vi "markReadOnly.vi"(8 "error in (no error)":errorcluster, 11 "Context in":T1) -> (0 "error out":errorcluster, 3 "Context out":T1)   [LabVIEW 2022 SP3, in "Property Editor.lvlib"]
uses:
  Property Editor.lvlib
  Public/Classes/IComponent/IComponent.lvclass
  TypeDef/DisplayType.ctl
  TypeDef/Context.ctl
  Public/Classes/IProperty/IProperty.lvclass
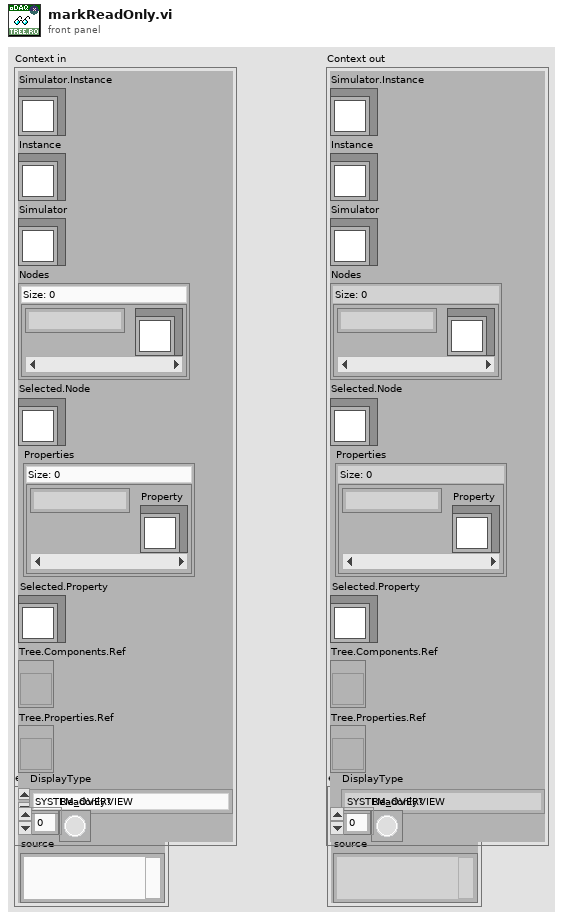
[diagram p1: front panel]
types:
  T1 = typedef "Property Editor.lvlib/Context.ctl" = cluster{"Simulator.Instance":refnum<class "IComponent.lvclass">, "Instance":refnum<class "IComponent.lvclass">, "Simulator":refnum<class "IComponent.lvclass">, "Nodes":map{string, refnum<class "IComponent.lvclass">}, "Selected.Node":refnum<class "IComponent.lvclass">, "Properties":map{string, refnum<class "IProperty.lvclass">}, "Selected.Property":refnum<class "IProperty.lvclass">, "Tree.Components.Ref":refnum<vi>, "Tree.Properties.Ref":refnum<vi>, "DisplayType":T2, "Readonly?":bool[]}
  T2 = typedef "Property Editor.lvlib/DisplayType.ctl" = enum16{"SYSTEM_OVERVIEW", "SIGNALS", "CHANNELS", "FUNCTION_BLOCKS", "TOPOLOGY", "TOPOLOGY_CUSTOM_COMPONENTS", "UNSPECIFIED"}
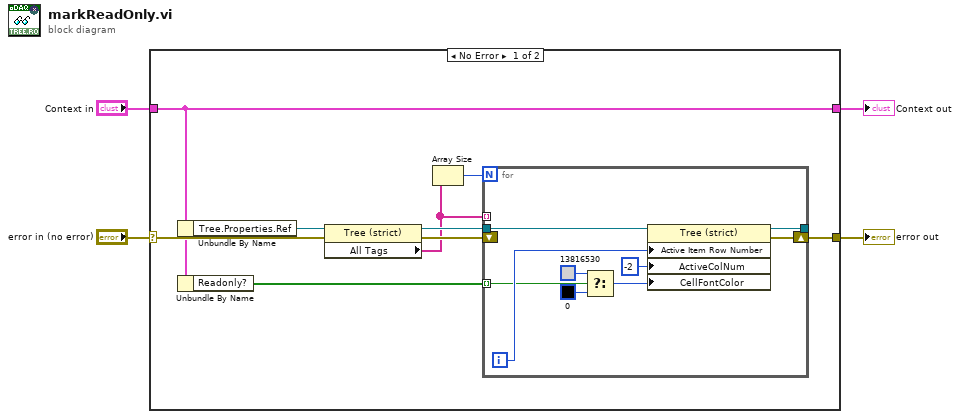
[diagram p0: block diagram]
diagram:
  n1 = case shown="No Error" "error in (no error)" {
    selector: "error in (no error)" -> [w8 w24]
    tunnel: [w13 w24] -> w4
    tunnel: "Context in" -> [w5 w23]
    tunnel: [w5 w23] -> w1
    frame No Error {
      n2 = Unbundle By Name(w5) -> ("Tree.Properties.Ref"=w7:refnum<vi>)
      n3 = Unbundle By Name(w5) -> ("Readonly?"=w6:bool[])
      n4 = property class="Tree (strict)"(reference=w7, error in=w8) -> (reference out=w11:refnum<vi>, error out=w12:errorcluster, "All Tags"=w10:string[])
      n5 = Array Size(array=w10) -> (size(s)=w9:i32)
      n6 = for {
        N: w9 -> [_]
        tunnel: w11 -> [w21]
        tunnel: w10 -> [_] mode=indexing
        tunnel: [w16] -> _
        shift-right: [w15] -> w13
        shift-left: w12 -> [_]
        tunnel: w6 -> [w14] mode=indexing
        i -> [w20]
        n7 = Select(t=u32 13816530 ("Active Cell:Cell Font:Color"), s=w14, f=u32 0 ("Active Cell:Cell Font:Color")) -> (s? t:f=w17:u32)
        n8 = property class="Tree (strict)"(reference=w21, "Active Item Row Number"=w20, "ActiveColNum"=-2 ("Active Cell:Active Column Number"), "CellFontColor"=w17) -> (reference out=w16:refnum<vi>, error out=w15:errorcluster)  [unwired: 1 in]
      }
    }
    frame Error {
    }
  }
  "error out" <- w4
  "Context out" <- w1
